vi "Set API  Token.vi"(7 "Persist?":bool, 8 "error in (no error)":errorcluster, 10 "Token":string, 11 "REST Client in":refnum<class "REST Client.lvclass">) -> (0 "error out":errorcluster, 3 "REST Client out":refnum<class "REST Client.lvclass">)   [LabVIEW 2024, in "ETL API.lvlib"]
uses:
  ETL API.lvlib
  <vilib>/addons/_JKI.lib/REST Client/classes/REST Client/REST Client.lvclass
  <vilib>/addons/_JKI.lib/REST Client/classes/REST Client/HTTP Header.ctl
  <vilib>/NI/Advanced HTTP Client/Header--Combo Box.ctl
  <vilib>/NI/Advanced HTTP Client/Session.lvclass
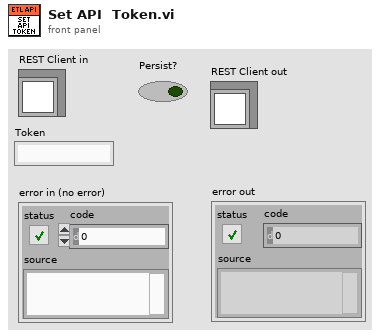
[diagram p1: front panel]
types:
  T1 = typedef "lib_NI_Advanced HTTP Client.lvlib/Session.lvclass/Header--Combo Box.ctl" = string
  T2 = typedef "REST Client.lvlib/REST Client.lvclass/HTTP Header.ctl" = cluster{"header":T1, "value":string}
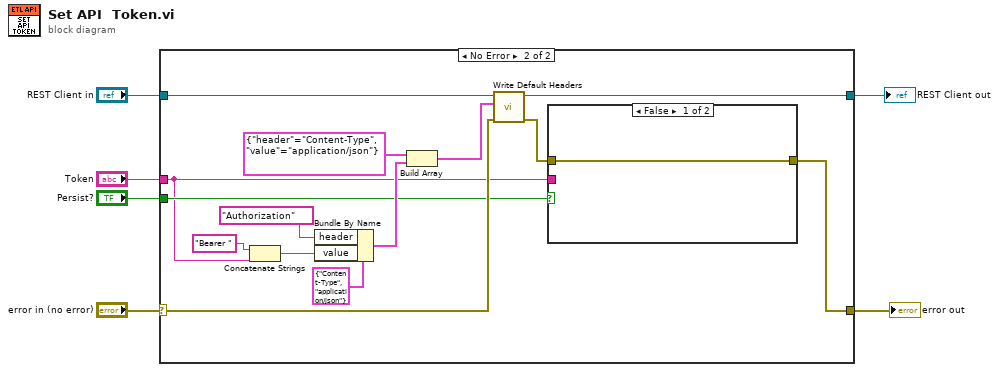
[diagram p0: block diagram]
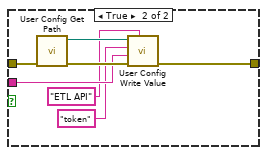
[diagram p3: hidden frame]
diagram:
  n1 = case shown="No Error" "error in (no error)" {
    selector: "error in (no error)" -> [w8 w14]
    tunnel: [w8 w9] -> w5
    tunnel: "Token" -> [_ w10]
    tunnel: "REST Client in" -> [w7 w16]
    tunnel: [w7 w11] -> w2
    tunnel: "Persist?" -> [_ w13]
    frame Error {
    }
    frame No Error {
      n2 = Concatenate Strings("Bearer " ("string"), w10) -> (w18:string)
      n3 = Bundle By Name(cluster=T2 {"header"="Content-Type", "value"="application/json"} ("Header"), "header"=T1 "Authorization", "value"=w18) -> (w17:T2)
      n4 = Build Array(T2 {"header"="Content-Type", "value"="application/json"} ("Header"), w17) -> (w15:T2[])
      n5 = call-dynamic "Write Default Headers.vi"("error in (no error)"=w14, "Headers"=w15, "REST Client in"=w16) -> ("error out"=w12:errorcluster, "REST Client out"=w11:refnum<class "REST Client.lvclass">)  [unwired: 7 in]
      n6 = case shown="False" w13 {
        tunnel: w12 -> [w23 w28]
        tunnel: w10 -> [_ w27]
        tunnel: [w23 w24] -> w9
        frame False {
        }
        frame True {
          n7 = call "User Config Get Path.vi"("error in (no error)"=w28) -> ("error out"=w30:errorcluster, "INI Path"=w29:path)  [unwired: 9 in]
          n8 = call "User Config Write Value.vi"("Section"="ETL API", "error in (no error)"=w30, "Value"=w27, "Key"="token", "INI File Path"=w29) -> ("error out"=w24:errorcluster)  [unwired: 4 in, 2 out]
        }
      }
    }
  }
  "error out" <- w5
  "REST Client out" <- w2
